vi "ChannelSelectionScreen.vi"(7 "Generate?":bool, 8 "error in":errorcluster, 10 "Frame Configuration":T1 {"CRC"."Data Type" items=["Signed", "Unsigned", "IEEE Float"]; "Rolling Counter"."Data Type" items=["Signed", "Unsigned", "IEEE Float"]; "Input Channels"."Data Type" items=["Signed", "Unsigned", "IEEE Float"]}, 11 "Parent Ref":T4=18446744073709551615 format="%.0x") -> (0 "error out":errorcluster, 1 "Cancelled?":bool, 2 "Frame Configuration out":T1 {"CRC"."Data Type" items=["Signed", "Unsigned", "IEEE Float"]; "Rolling Counter"."Data Type" items=["Signed", "Unsigned", "IEEE Float"]; "Input Channels"."Data Type" items=["Signed", "Unsigned", "IEEE Float"]}, 3 "Parent Ref Out":T4=18446744073709551615 format="%.0x")   [LabVIEW 2016, in "LIN Frame Protection Addon System Explorer.lvlib"]
uses:
  LIN Frame Protection Addon System Explorer.lvlib
  NationalInstruments.VeriStand.SystemStorageUI
  <vilib>/NI Veristand/Custom Device API/Custom Device Item Ref.ctl
  Shared/Types/FrameConfiguration.ctl
  Shared/Types/InputChannelConfiguration.ctl
  Shared/Types/Protection Type.ctl
  <vilib>/NI Veristand/Custom Device API/Custom Device API.lvlib
  <vilib>/NI Veristand/Custom Device Tools/Custom Device Utility Library/Custom Device Utility Library.lvlib
  Shared/LIN Frame Protection Addon Shared.lvlib
panel:
  in  "Max Count":dbl=4.0
  in  "Rolling Counter":refnum<k24>(container)
  in  "Protection":refnum<k24>(container)
  in  "Cancel":bool
  in  "OK":bool
  in  "Protection Data":refnum<k24>(container)
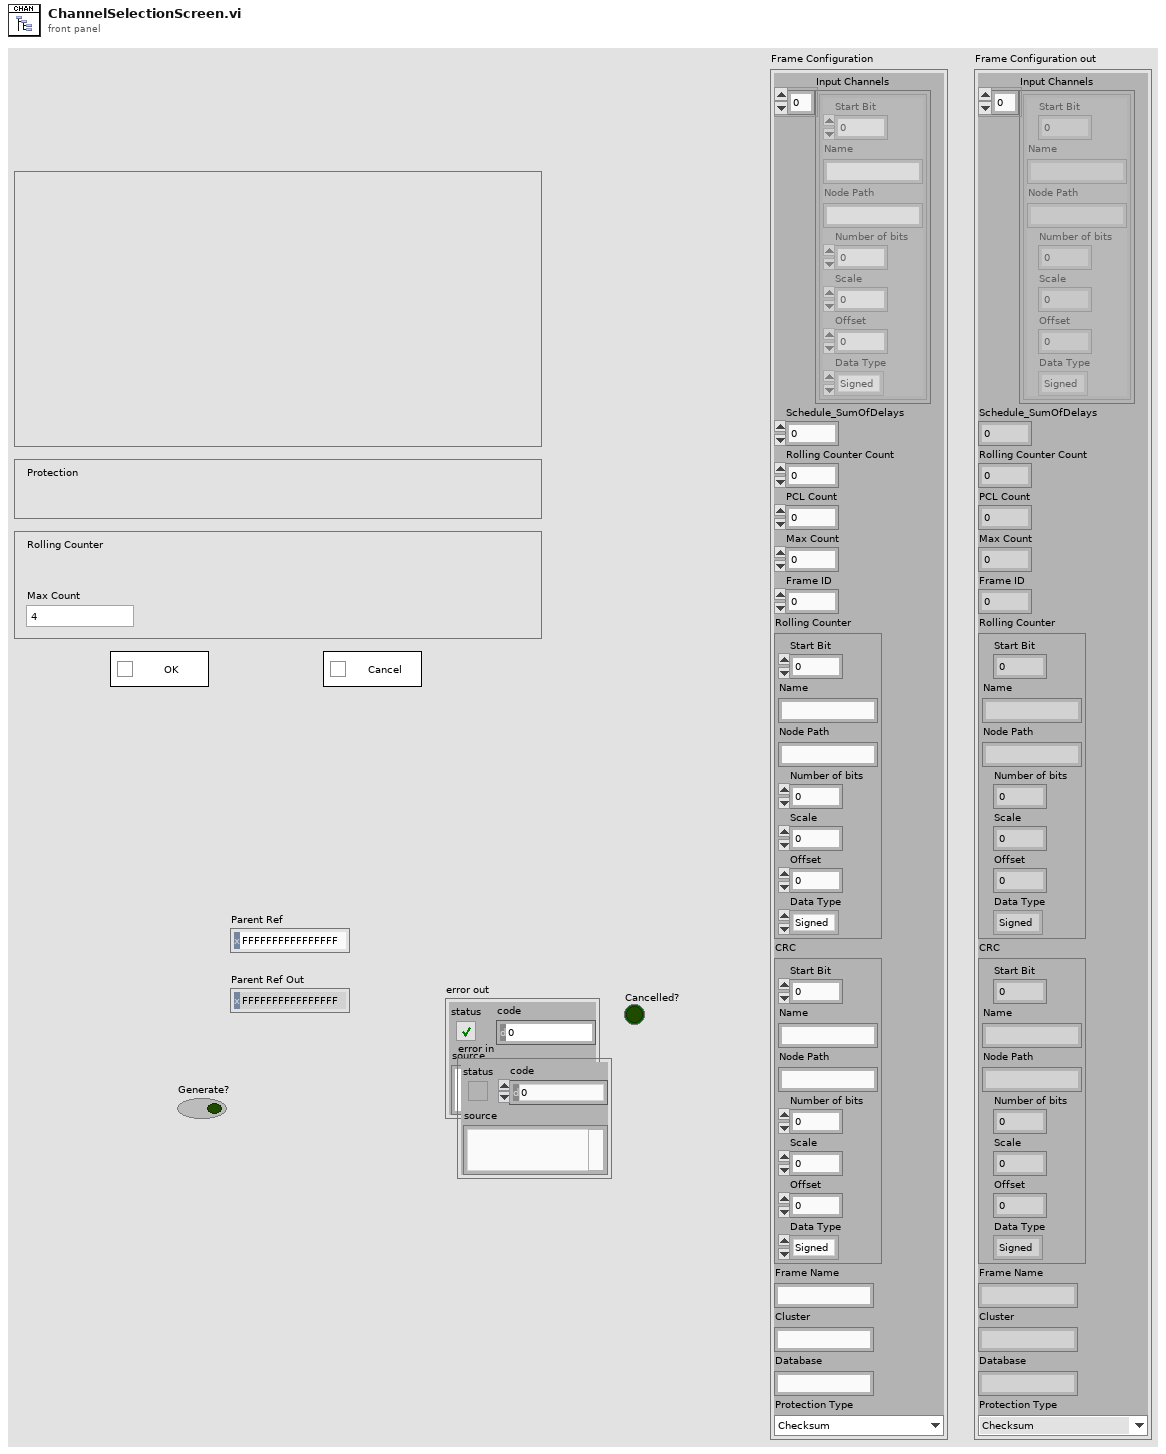
[diagram p1: front panel]
types:
  T1 = typedef "LIN Frame Protection Addon Shared.lvlib/FrameConfiguration.ctl" = cluster{"Input Channels":T2[], "Schedule_SumOfDelays":dbl, "Rolling Counter Count":dbl, "PCL Count":u64, "Max Count":dbl, "Frame ID":u32, "Rolling Counter":T2, "CRC":T2, "Frame Name":string, "Cluster":string, "Database":string, "Protection Type":T3}
  T2 = typedef "LIN Frame Protection Addon Shared.lvlib/InputChannelConfiguration.ctl" = cluster{"Start Bit":i32, "Name":string, "Node Path":string, "Number of bits":i32, "Scale":dbl, "Offset":dbl, "Data Type":u32}
  T3 = typedef "LIN Frame Protection Addon Shared.lvlib/Protection Type.ctl" = enum16{"Checksum", "CRC", "None (Counter Only)"}
  T4 = typedef "Custom Device API.lvlib/Custom Device Item Ref.ctl" = u64
  T5 = typedef "Custom Device API.lvlib/Custom Device Pointer.ctl" = refnum<k24>
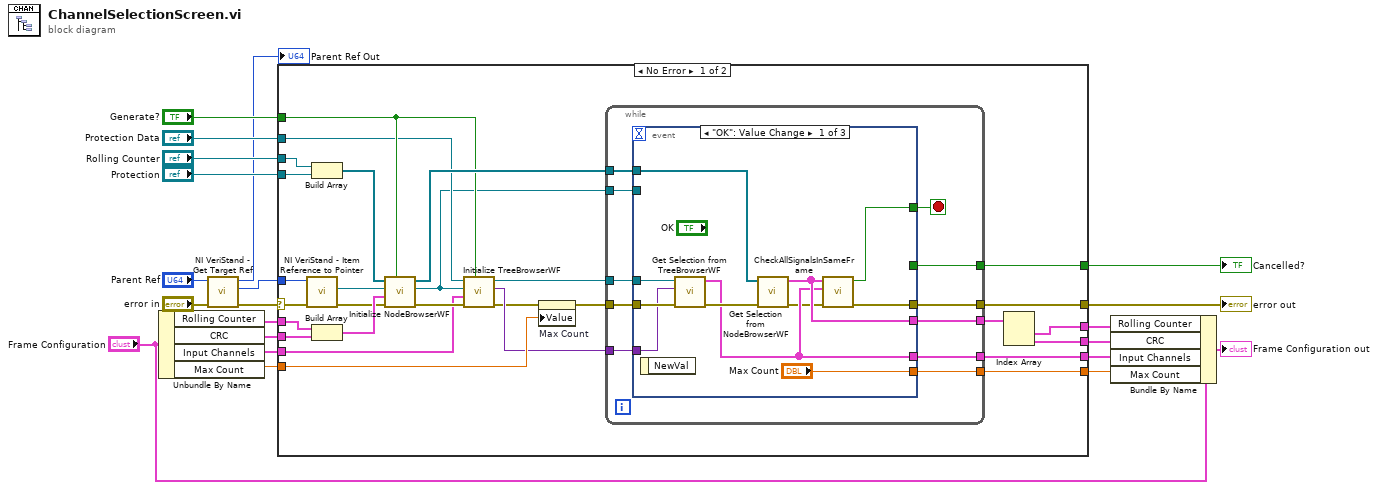
[diagram p0: block diagram]
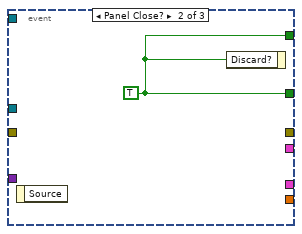
[diagram p2: hidden frame]
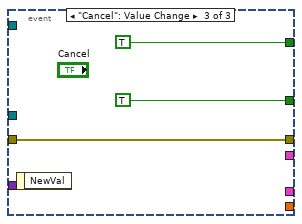
[diagram p3: hidden frame]
diagram:
  n1 = Unbundle By Name("Frame Configuration") -> ("Rolling Counter"=w9:T2, "CRC"=w8:T2, "Input Channels"=w15:T2[], "Max Count"=w4:dbl)
  n2 = call <vilib>:"NI VeriStand - Get Target Ref.vi"("error in"="error in", "Item Ref in"="Parent Ref") -> ("error out"=w17:errorcluster, "Target Ref"=w1:T4, "Item Ref out"=→"Parent Ref Out":T4)  [unwired: 6 in, 1 out]
  n3 = case shown="No Error" w17 {
    selector: w17 -> [w48 w76]
    tunnel: "Protection Data" -> [w28 _]
    tunnel: w1 -> [w49 _]
    tunnel: [w47 _] -> w20
    tunnel: [w22 w76] -> w19
    tunnel: [w46 _] -> w14
    tunnel: w15 -> [w37 _]
    tunnel: "Rolling Counter" -> [w44 _]
    tunnel: "Protection" -> [w45 _]
    tunnel: w9 -> [w43 _]
    tunnel: w8 -> [w42 _]
    tunnel: [w34 _] -> w7
    tunnel: [w33 _] -> w6
    tunnel: [w32 _] -> w5
    tunnel: w4 -> [w30 _]
    tunnel: "Generate?" -> [w29 _]
    frame No Error {
      n4 = call <vilib>:"NI VeriStand - Item Reference to Pointer.vi"("error in (no error)"=w48, "Item Ref in"=w49) -> ("error out"=w40:errorcluster, "Node Pointer"=w27:T5)  [unwired: 6 in, 2 out]
      n5 = Build Array(w44, w45) -> (w38:refnum<k24>[])
      n6 = Build Array(w43, w42) -> (w41:T2[])
      n7 = call "Initialize NodeBrowserWF.vi"("Generate?"=w29, "error in (no error)"=w40, "Output Channels"=w41, "Node Pointer"=w27, "NodeBrowserRefs"=w38) -> ("error out"=w39:errorcluster, "Node Pointer"=w25:T5, "NodeBrowserRefs"=w36:refnum<k24>[])  [unwired: 4 in]
      n8 = call "Initialize TreeBrowserWF.vi"("Generate?"=w29, "error in (no error)"=w39, "Input Channels"=w37, "Node Pointer"=w25, "TreeBrowserRef"=w28) -> ("error out"=w23:errorcluster, "Channels"=w26:variant, "TreeBrowserRef 2"=w24:refnum<k24>)  [unwired: 4 in]
      n9 = property on="Max Count" class="DigNum (strict)"(error in=w23, "Value"=w30) -> (error out=w31:errorcluster)  [unwired: 1 in, 1 out]
      n10 = while {
        tunnel: w31 -> [w60]
        tunnel: w24 -> [w59]
        tunnel: [w57] -> w47
        tunnel: [w56] -> w22
        tunnel: [w55] -> w46
        tunnel: w26 -> [w54]
        tunnel: w36 -> [w53]
        tunnel: [w52] -> w35
        tunnel: [w51] -> w32
        tunnel: w25 -> [w50]
        stop <- w58 stop-if-true
        n11 = event shown="[0] \"OK\": Value Change" {
          selector: _ -> [_ _ _]
          dyn-events: _ -> [_ _ _]
          timeout: _ -> [_ _ _]
          tunnel: w60 -> [w71 _ w75]
          tunnel: w59 -> [w70 _ _]
          tunnel: [w63 _ w75] -> w56
          tunnel: [w62 w72 TRUE] -> w58
          tunnel: [_ w72 TRUE] -> w57
          tunnel: [w65 _ _] -> w55
          tunnel: w54 -> [w69 _ _]
          tunnel: w53 -> [w68 _ _]
          tunnel: [w66 _ _] -> w52
          tunnel: ["Max Count" _ _] -> w51
          tunnel: w50 -> [_ _ _]
          event "OK": Value Change {
            n12 = event-data() -> ()  [unwired: 1 in, 1 out]
            n13 = call "Get Selection from TreeBrowserWF.vi"("error in (no error)"=w71, "Input Channels"=w69, ".NET Refnum in"=w70) -> ("error out"=w67:errorcluster, "Input Channel Selections"=w65:T2[])  [unwired: 7 in]
            n14 = call "Get Selection from NodeBrowserWF.vi"("error in (no error)"=w67, "NodeBrowserRefs"=w68) -> ("error out"=w64:errorcluster, "Array"=w66:T2[])  [unwired: 8 in]
            n15 = call "CheckAllSignalsInSameFrame.vi"("error in"=w64, "Input Channel Selections"=w65, "Rolling Counter and CRC"=w66) -> ("error out"=w63:errorcluster, "Pass?"=w62:bool)  [unwired: 7 in]
          }
          event Panel Close? {
            w72 = TRUE
            n16 = event-data() -> ()  [unwired: 1 in, 1 out]
            n17 = event-data("Discard?"=w72) -> ()  [unwired: 1 in, 1 out]
          }
          event "Cancel": Value Change {
            n18 = event-data() -> ()  [unwired: 1 in, 1 out]
          }
        }
      }
      n19 = Index Array(array=w35) -> (element #1=w33:T2, element #2=w34:T2)  [unwired: 2 in]
    }
    frame Error {
    }
  }
  "Cancelled?" <- w20
  "error out" <- w19
  n20 = Bundle By Name(cluster="Frame Configuration", "Rolling Counter"=w6, "CRC"=w7, "Input Channels"=w14, "Max Count"=w5) -> (→"Frame Configuration out":T1)
